vi "Get Groups In Memory.vi"(8 "error in (no error)":errorcluster) -> (0 "error out":errorcluster, 3 "Groups In Memory":T1[](array[typedef]))   [LabVIEW 2020, in "Current Value Table(Rebuild).lvlib"]
doc: "This VI retrieves all groups in memory and the tags associated with them."
uses:
  Type Defs/Tag Grouping set.ctl
  FGVs/Group Memory Methods.ctl
  Current Value Table(Rebuild).lvlib
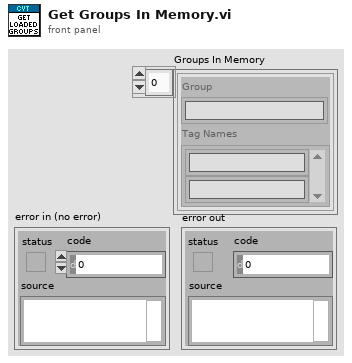
[diagram p1: front panel]
types:
  T1 = typedef "Current Value Table(Rebuild).lvlib/Tag Grouping set.ctl" = cluster{"Group":string, "Tag Names":string[]}
  T2 = typedef "Current Value Table(Rebuild).lvlib/Group Memory Methods.ctl" = enum16{"Clear", "Read Indices in Group", "List Groups", "List Tags by Type", "List Tags", "Delete Group", "Check Group Existence", "Create Group"}
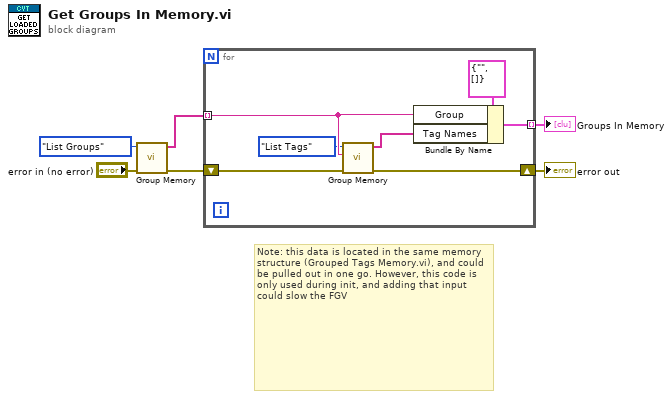
[diagram p0: block diagram]
diagram:
  # "Note: this data is located in the same memory structure (Grouped Tags Memory.vi), and could be pulled out in one go. However, this code is only used during init, and adding that input could slow the FGV"
  n1 = call "Group Memory.vi"("error in (no error)"="error in (no error)", "Method"=Group_Memory_Methods."List Groups") -> ("error out"=w5:errorcluster, "Tags/Groups Out"=w6:string[])  [unwired: 6 in, 2 out]
  n2 = for {
    shift-right: [w10] -> w2
    shift-left: w5 -> [w11]
    tunnel: [w12] -> w4 mode=indexing
    tunnel: w6 -> [w9] mode=indexing
    n3 = call "Group Memory.vi"("error in (no error)"=w11, "Group"=w9, "Method"=Group_Memory_Methods."List Tags") -> ("error out"=w10:errorcluster, "Tags/Groups Out"=w8:string[])  [unwired: 5 in, 2 out]
    n4 = Bundle By Name(cluster=T1 {"Group"="", "Tag Names"=[]} ("Tag Grouping"), "Group"=w9, "Tag Names"=w8) -> (w12:T1)
  }
  "Groups In Memory" <- w4
  "error out" <- w2
